vi "Write Nickname.vi"(8 "error in (no error)":errorcluster, 10 "Nickname":string, 11 "Pele in":refnum<class "Pele.lvclass">) -> (0 "error out":errorcluster, 3 "Pele out":refnum<class "Pele.lvclass">)   [LabVIEW 2019, in "Pele.lvclass"]
uses:
  Pele.lvclass
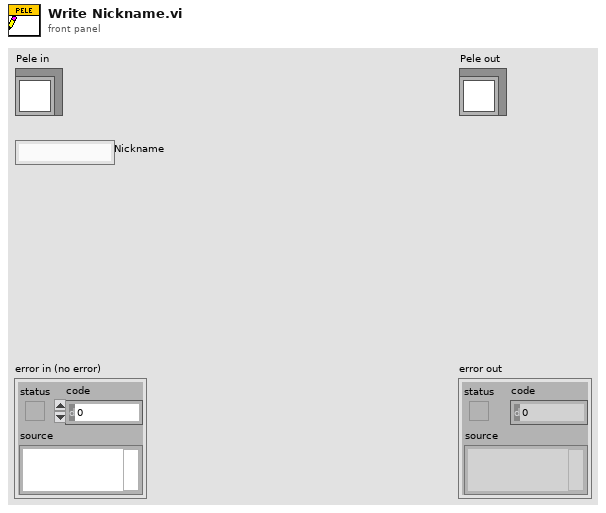
[diagram p1: front panel]
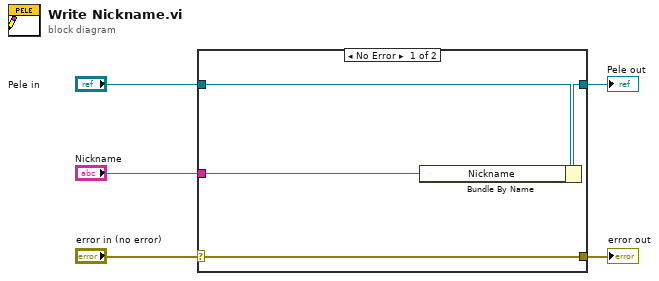
[diagram p0: block diagram]
diagram:
  n1 = case shown="No Error" "error in (no error)" {
    selector: "error in (no error)" -> [w9 w10]
    tunnel: [w9 w10] -> w4
    tunnel: [w7 w11] -> w2
    tunnel: "Pele in" -> [w8 w11]
    tunnel: "Nickname" -> [w6 _]
    frame No Error {
      n2 = Bundle By Name(cluster=w8, "Nickname"=w6) -> (w7:refnum<class "Pele.lvclass">)
    }
    frame Error {
    }
  }
  "error out" <- w4
  "Pele out" <- w2
